vi "CalculatePowerPursuit.vi"(6 "Reset":bool, 9 "Gains":T1={"FFV"=0.01, "FFA"=0.01, "Vel PID"={"P"=0.01, "I"=0.0, "D"=0.0}} {"Vel PID"."D" format="%.3f"; "Vel PID"."I" format="%.3f"; "Vel PID"."P" format="%.3f"}, 10 "Vel":dbl, 11 "Target Vel":dbl) -> (3 "Power":dbl)   [LabVIEW 2017]
doc: "Uses a PIDF controller to achieve target velocity for each wheel.\n\nMaybe we could break this VI out into another loop so we could run it faster than 20ms?"
uses:
  <vilib>/addons/control/pid/pid.llb/PID (DBL).vi
  <vilib>/addons/control/pid/NI_PID_pid.lvlib
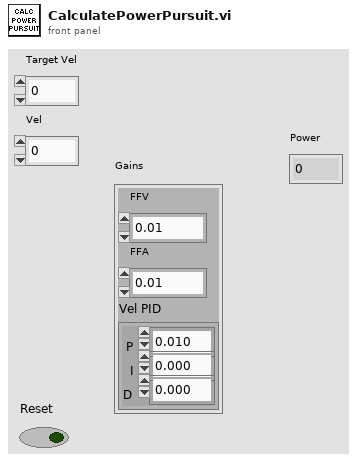
[diagram p1: front panel]
types:
  T1 = cluster{"FFV":dbl, "FFA":dbl, "Vel PID":cluster{"P":dbl, "I":dbl, "D":dbl}}
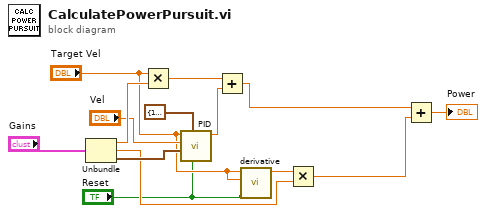
[diagram p0: block diagram]
diagram:
  n1 = Unbundle("Gains") -> ("FFV"=w14:dbl, "FFA"=w6:dbl, "Vel PID"=w7:cluster{"P":dbl, "I":dbl, "D":dbl})
  n2 = Multiply(x="Target Vel", y=w14) -> (x*y=w12:dbl)
  n3 = call-poly <vilib>:"PID.vi"("reinitialize? (F)"="Reset", "output range"=cluster{"output high":dbl, "output low":dbl} {"output high"=1.0, "output low"=-1.0}, "PID gains"=w7, "process variable"="Vel", "setpoint"="Target Vel") -> ("output"=w11:dbl)  [unwired: 5 in, 1 out]
  n4 = Add(x=w12, y=w11) -> (x+y=w5:dbl)
  n5 = call "derivative.vi"("Reset"="Reset", "Starting value"="Target Vel", "x"="Target Vel") -> ("dx/dt"=w9:dbl)  [unwired: 8 in]
  n6 = Multiply(x=w9, y=w6) -> (x*y=w4:dbl)
  n7 = Add(x=w5, y=w4) -> (x+y=→"Power":dbl)
